vi "3d point cloud display.vi"() -> ()   [LabVIEW 2009]
uses:
  <vilib>/Utility/miscctls.llb/LVRGBAColorTypeDef.ctl
  <vilib>/Utility/miscctls.llb/LV3DPointTypeDef.ctl
  <vilib>/picture/3D Picture Control/NI_3D Picture Control.lvlib
panel:
  in  "file path (dialog if empty)":path
  in  "From File?":bool
  in  "Camera Controller:Type":T1(ring)=enum."Spherical"
  in  "stop":bool
  out "3D Picture":refnum<vi>(3d-picture)
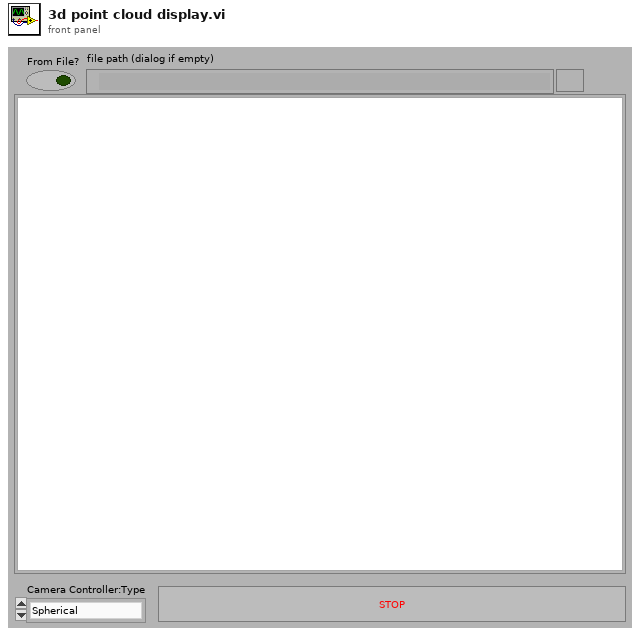
[diagram p1: front panel]
types:
  T1 = enum16{"None", "Spherical", "Flying", "Oriented"}
  T2 = typedef "LVRGBAColorTypeDef.ctl" = cluster{"Red":sgl, "Green":sgl, "Blue":sgl, "Alpha":sgl}
  T3 = enum16{"Overall", "Per Primitive", "Per Vertex", "Binding Off"}
  T4 = enum16{"Points", "Lines", "Line Strip", "Line Loop", "Triangles", "Triangle Strip", "Triangle Fan", "Quads", "Quad Strip", "Polygon"}
  T5 = typedef "LV3DPointTypeDef.ctl" = cluster{"X":sgl, "Y":sgl, "Z":sgl}
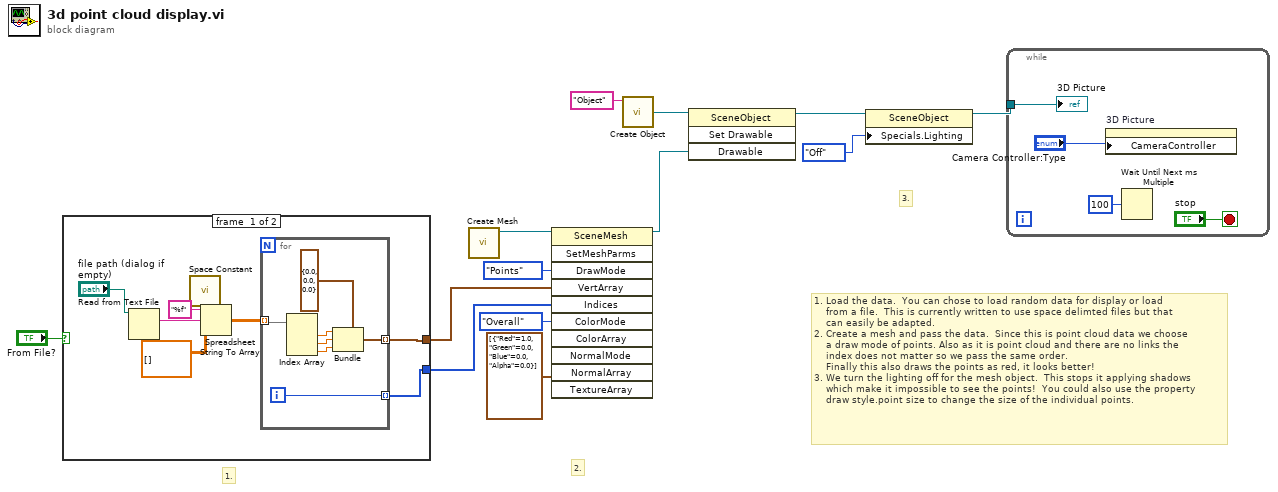
[diagram p0: block diagram]
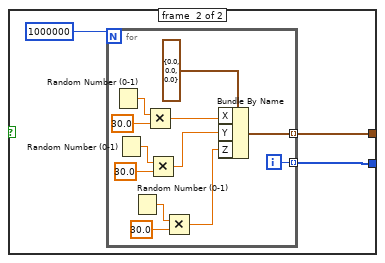
[diagram p2: hidden frame]
diagram:
  # "1. Load the data.  You can chose to load random data for display or load \n    from a file.  This is currently written to use space delimted files but that\n    can easily be adapted.\n2. Create a mesh and pass the data.  Since this is point cloud data we choose\n    a draw mode of points. Also as it is point cloud and there are no links the \n    index does not matter so we pass the same order.\n    Finally this also draws the points as red, it looks better!\n3. We turn the lighting off for the mesh object.  This stops it applying shadows\n    which make it impossible to see the points!  You could also use the property\n    draw style.point size to change the size of the individual points."
  # "3."
  # "2."
  # "1."
  n1 = case shown="False" "From File?" {
    tunnel: [w15 w30] -> w11
    tunnel: [w14 w29] -> w1
    frame #0 {
      n2 = Read from Text File(file (use dialog)="file path (dialog if empty)") -> (text=w20:string)  [unwired: 3 in, 3 out]
      n3 = call <vilib>:"Space Constant.vi"() -> ("String"=w19:string)
      n4 = Spreadsheet String To Array(delimiter (Tab)=w19, format string="%f", spreadsheet string=w20, array type (2D Dbl)=sgl[][] []) -> (array=w17:sgl[][])
      n5 = for {
        tunnel: w17 -> [w28] mode=indexing
        tunnel: [w23] -> w15 mode=indexing
        tunnel: [w22] -> w14 mode=indexing
        i -> [w22]
        n6 = Index Array(array=w28) -> (element #1=w26:sgl, element #2=w25:sgl, element #3=w24:sgl)  [unwired: 3 in]
        n7 = Bundle(cluster=T5 {"X"=0.0, "Y"=0.0, "Z"=0.0} ("3D Point"), "X"=w26, "Y"=w25, "Z"=w24) -> (w23:T5)
      }
    }
    frame #1 {
      n8 = for {
        N: 1000000 -> [_]
        tunnel: [w33] -> w30 mode=indexing
        tunnel: [w32] -> w29 mode=indexing
        i -> [w32]
        n9 = Random Number (0-1)() -> (number: 0 to 1=w41:dbl)
        n10 = Random Number (0-1)() -> (number: 0 to 1=w40:dbl)
        n11 = Random Number (0-1)() -> (number: 0 to 1=w37:dbl)
        n12 = Multiply(x=w41, y=30.0) -> (x*y=w36:dbl)
        n13 = Multiply(x=w40, y=30.0) -> (x*y=w35:dbl)
        n14 = Multiply(x=w37, y=30.0) -> (x*y=w34:dbl)
        n15 = Bundle By Name(cluster=T5 {"X"=0.0, "Y"=0.0, "Z"=0.0} ("3D Point"), "X"=w36, "Y"=w35, "Z"=w34) -> (w33:T5)
      }
    }
  }
  n16 = call <vilib>:"Create Mesh.vi"() -> ("New Mesh Refnum"=w9:refnum<vi>)  [unwired: 10 in, 1 out]
  n17 = invoke class="SceneMesh" method="SetMeshParms"(reference=w9, "DrawMode"=T4."Points" ("Draw Mode"), "VertArray"=w11, "Indices"=w1, "ColorMode"=T3."Overall" ("Color Binding Mode"), "ColorArray"=T2[] [{"Red"=1.0, "Green"=0.0, "Blue"=0.0, "Alpha"=0.0}] ("Color Array")) -> (reference out=w5:refnum<vi>)  [unwired: 5 in, 10 out]
  n18 = call <vilib>:"Create Object.vi"("Name"="Object") -> ("Scene:New Object"=w12:refnum<vi>)  [unwired: 9 in, 1 out]
  n19 = invoke class="SceneObject" method="Set Drawable"(reference=w12, "Drawable"=w5) -> (reference out=w4:refnum<vi>)  [unwired: 2 in, 3 out]
  n20 = property class="SceneObject"(reference=w4, "Specials.Lighting"=enum16{"Inherit Value", "Off", "On"}."Off" ("Specials:Lighting")) -> (reference out=w3:refnum<vi>)  [unwired: 1 in, 1 out]
  n21 = while {
    tunnel: w3 -> [w47]
    stop <- "stop" stop-if-true
    n22 = property on="3D Picture" class="SceneGraphDisp (strict)"("CameraController"="Camera Controller:Type") -> ()  [unwired: 2 in, 2 out]
    n23 = Wait Until Next ms Multiple(millisecond multiple=u32 100) -> ()  [unwired: 1 out]
    "3D Picture" <- w47
  }
